vi "Copy Image (ARGB with Greyscale Mask).vi"(8 "error in (no error)":errorcluster, 9 "Greyscale Image Mask":T1, 10 "ARGB Image Destination":T2, 11 "ARGB Image Source":T2) -> (0 "error out":errorcluster, 3 "ARGB Image Destination (duplicate)":T2)   [LabVIEW 2020, in "g_ar_toolkit.image.lvlib"]
uses:
  g_ar_toolkit.image.lvlib
  ARGB Image.ctl
  Greyscale Image.ctl
  327a14ae-2acc-4952-87c0-fab6c3cd3da3.vi
  g_ar_toolkit.common/Module Path.vi
  <vilib>/Utility/error.llb/Error Cluster From Error Code.vi
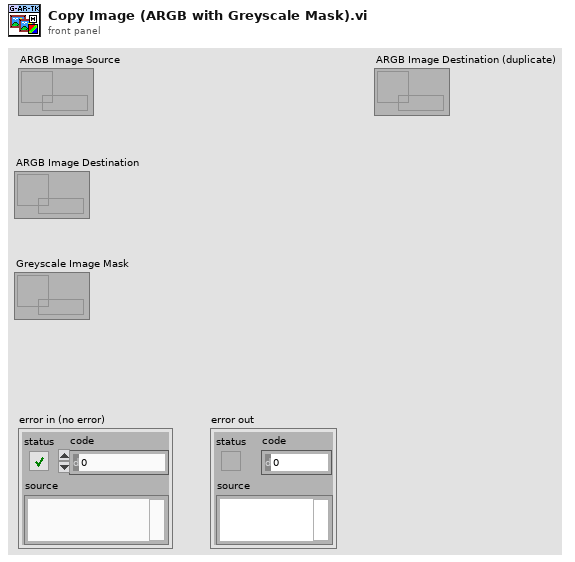
[diagram p1: front panel]
types:
  T1 = typedef "g_ar_toolkit.image.lvlib/Greyscale Image.ctl" = refnum<data-value>
  T2 = typedef "g_ar_toolkit.image.lvlib/ARGB Image.ctl" = refnum<data-value>
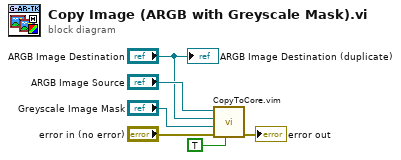
[diagram p0: block diagram]
diagram:
  n1 = call "CopyToCore.vim"("Has Mask"=TRUE, "error in (no error)"="error in (no error)", "Mask"="Greyscale Image Mask", "Dst"="ARGB Image Destination", "Src"="ARGB Image Source") -> ("error out"=→"error out":errorcluster)  [unwired: 6 in]
  "ARGB Image Destination (duplicate)" <- "ARGB Image Destination"
